vi "Parse Library References for Documentable Types.vi"(7 "Config":refnum<class "TAF Proj Config.lvclass">, 8 "error in":errorcluster, 10 "VI References":refnum<vi>[](array[refnum]), 11 "Library References":refnum<vi>[](array[refnum])) -> (0 "error out":errorcluster, 3 "Blocs":T1)   [LabVIEW 2021, in "TAF Proj Document Type.lvlib" / "Project Parser.lvlib"]
doc: "Iterates through all <b>Library References</b> and parses the following types:\n- DQMH Modules\n- Other Libraries\n- LVClasses"
uses:
  <vilib>/Wovalab/AntiDoc/Document Type/Add-ons/LabVIEW TAF Project/Project Parser/Project Parser.lvlib
  <vilib>/Wovalab/AntiDoc/Document Type/Add-ons/LabVIEW TAF Project/Project Parser/Blocs--cluster.ctl
  <vilib>/Wovalab/AntiDoc/Document Type/Add-ons/LabVIEW TAF Project/Custom Errors/Custom Errors.lvclass
  <vilib>/Wovalab/AntiDoc/Document Type/Add-ons/LabVIEW TAF Project/Classes Overview/Classes Overview.lvclass
  <vilib>/Wovalab/AntiDoc/Document Type/Add-ons/LabVIEW TAF Project/Dqmh Modules Overview/Dqmh Modules Overview.lvclass
  <vilib>/Wovalab/AntiDoc/Document Type/Add-ons/LabVIEW TAF Project/FrontPanelGUI/FrontPanelGUI.lvclass
  <vilib>/Wovalab/AntiDoc/Document Type/Add-ons/LabVIEW TAF Project/Dqmh Module/Dqmh Module.lvclass
  <vilib>/Wovalab/AntiDoc/Document Type/Add-ons/LabVIEW TAF Project/Class/Class.lvclass
  <vilib>/Wovalab/AntiDoc/Document Type/Add-ons/LabVIEW TAF Project/Lib/Lib.lvclass
  <vilib>/Wovalab/AntiDoc/Document Type/Add-ons/LabVIEW TAF Project/TAFConfiguration/TAFConfiguration.lvclass
  <vilib>/Wovalab/AntiDoc/Document Type/Add-ons/LabVIEW TAF Project/TAF Proj Config/TAF Proj Config.lvclass
  <vilib>/Wovalab/AntiDoc/Progress Bar/Progress Bar.lvlib
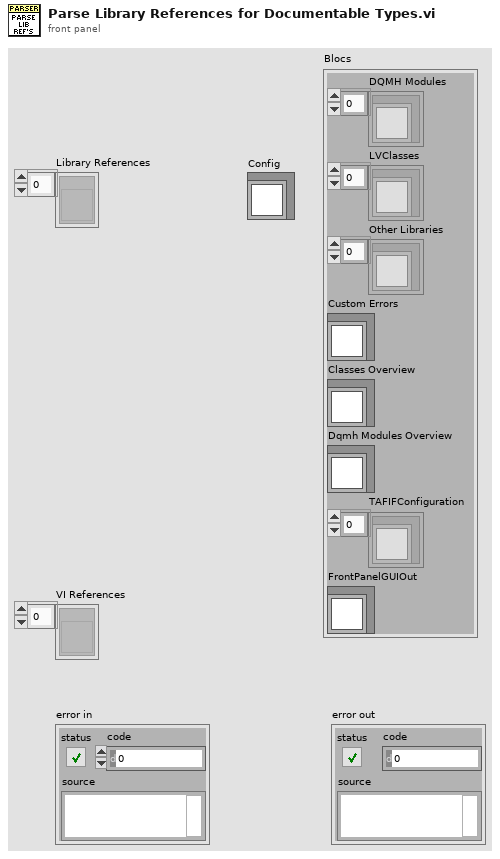
[diagram p1: front panel]
types:
  T1 = typedef "TAF Proj Document Type.lvlib/Project Parser.lvlib/Blocs--cluster.ctl" = cluster{"DQMH Modules":refnum<class "Dqmh Module.lvclass">[], "LVClasses":refnum<class "Class.lvclass">[], "Other Libraries":refnum<class "Lib.lvclass">[], "Custom Errors":refnum<class "Custom Errors.lvclass">, "Classes Overview":refnum<class "Classes Overview.lvclass">, "Dqmh Modules Overview":refnum<class "Dqmh Modules Overview.lvclass">, "TAFIFConfiguration":refnum<class "TAFConfiguration.lvclass">[], "FrontPanelGUIOut":refnum<class "FrontPanelGUI.lvclass">}
  T2 = typedef "TAF Proj Document Type.lvlib/Project Parser.lvlib/User Event Info.ctl" = cluster{"Vi Name":string, "User Event Names":string[]}
  T3 = typedef "TAF Proj Document Type.lvlib/Project Parser.lvlib/Custom Error Info.ctl" = cluster{"Code":i32, "Name":string, "Description":string, "Owned by":string}
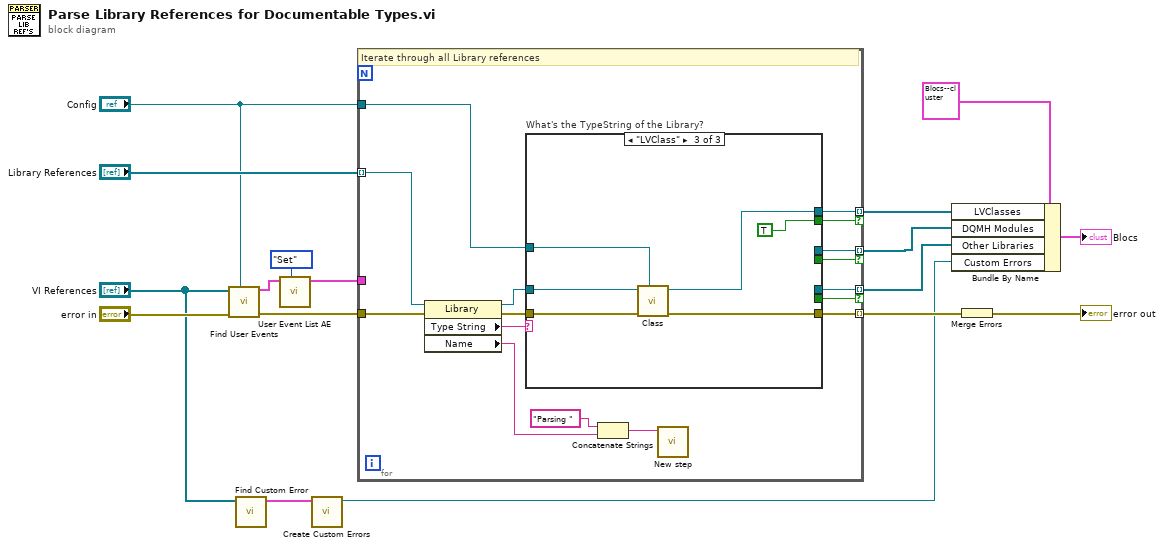
[diagram p0: block diagram]
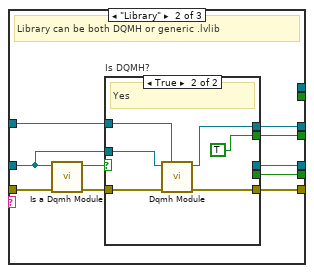
[diagram p3: hidden frame]
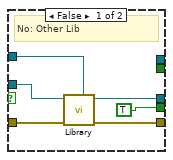
[diagram p4: hidden frame]
diagram:
  n1 = call <vilib>:"Find User Events.vi"("Config"="Config", "error in"="error in", "VI References"="VI References") -> ("error out"=w15:errorcluster, "User Event  Info"=w13:T2[])  [unwired: 7 in]
  n2 = call <vilib>:"Find Custom Error.vi"("VI References"="VI References") -> ("Custom Errors"=w11:T3[])  [unwired: 10 in]
  n3 = call <vilib>:"User Event List AE.vi"("Action"=enum16{"Set", "Get"}."Set", "Event Structure Info (set)"=w13) -> ("Event Structure Info Out"=w12:T2[])  [unwired: 9 in]
  n4 = call <vilib>:"Create Custom Errors.vi"("Custom Errors Info"=w11) -> ("Custom Errors out"=w6:refnum<class "Custom Errors.lvclass">)  [unwired: 9 in, 1 out]
  n5 = for {
    tunnel: [w30] -> w7 mode=indexing if=w29
    tunnel: [w33] -> w17 mode=indexing
    tunnel: "Library References" -> [w24] mode=indexing
    tunnel: [w28] -> w1 mode=indexing if=w27
    tunnel: w15 -> [w32]
    tunnel: [w26] -> w8 mode=indexing if=w25
    tunnel: w12 -> [_]
    tunnel: "Config" -> [w19]
    # "Iterate through all Library references"
    n6 = property class="Library"(reference=w24, error in=w32) -> (reference out=w23:refnum<vi>, error out=w31:errorcluster, "Type String"=w20:string, "Name"=w21:string)
    n7 = case "What's the TypeString of the Library?" shown="\"LVClass\"" w20 {
      tunnel: [_ w40 _] -> w30
      tunnel: [_ w43 w60] -> w33
      tunnel: w23 -> [_ w36 w58]
      tunnel: [_ w39 _] -> w29
      tunnel: [_ w38 _] -> w28
      tunnel: [_ w37 _] -> w27
      tunnel: [_ _ w57] -> w26
      tunnel: [_ _ TRUE] -> w25
      tunnel: w31 -> [_ w41 w61]
      tunnel: w19 -> [_ w34 w56]
      frame Default {
        # "Unknown or unsupported type"
      }
      frame "Library" {
        # "Library can be both DQMH or generic .lvlib"
        n8 = call <vilib>:"Is a Dqmh Module.vi"("error in"=w41, "Library Ref"=w36) -> ("error out"=w42:errorcluster, "Is Dqmh Module"=w35:bool)  [unwired: 7 in, 1 out]
        n9 = case "Is DQMH?" shown="True" w35 {
          tunnel: [w47 _] -> w40
          tunnel: [w49 w55] -> w43
          tunnel: w36 -> [w46 w53]
          tunnel: [TRUE _] -> w39
          tunnel: [_ w52] -> w38
          tunnel: [_ TRUE] -> w37
          tunnel: w42 -> [w48 w54]
          tunnel: w34 -> [w44 w50]
          frame False {
            # "No: Other Lib"
            n10 = call <vilib>:"Library.vi"("Config"=w44, "error in"=w48, "Library Ref"=w46) -> ("error out"=w49:errorcluster, "Lib out"=w47:refnum<class "Lib.lvclass">)  [unwired: 7 in]
          }
          frame True {
            # "Yes"
            n11 = call <vilib>:"Dqmh Module.vi"("Config"=w50, "error in (no error)"=w54, "Library Ref"=w53) -> ("error out"=w55:errorcluster, "Dqmh Module out"=w52:refnum<class "Dqmh Module.lvclass">)  [unwired: 7 in]
          }
        }
      }
      frame "LVClass" {
        n12 = call <vilib>:"Class.vi"("Config"=w56, "error in"=w61, "Library Ref"=w58) -> ("error out"=w60:errorcluster, "Class out"=w57:refnum<class "Class.lvclass">)  [unwired: 7 in]
      }
    }
    n13 = Concatenate Strings("Parsing " ("string"), w21) -> (w18:string)
    n14 = call <vilib>:"New step.vi"("Description"=w18) -> ()  [unwired: 10 in, 1 out]
  }
  n15 = Bundle By Name(cluster=T1 {"DQMH Modules"=[], "LVClasses"=[], "Other Libraries"=[], "Custom Errors"=refnum, "Classes Overview"=refnum, "Dqmh Modules Overview"=refnum, "TAFIFConfiguration"=[], "FrontPanelGUIOut"=refnum} ("Blocs"), "LVClasses"=w8, "DQMH Modules"=w1, "Other Libraries"=w7, "Custom Errors"=w6) -> (→"Blocs":T1)
  n16 = Merge Errors(w17) -> (→"error out":errorcluster)
